vi "Write Pixel Step.vi"(8 "error in (no error)":errorcluster, 10 "Pixel Step":i32, 11 "Listbox Handler in":refnum<class "Listbox Handler.lvclass">) -> (0 "error out":errorcluster, 3 "Listbox Handler out":refnum<class "Listbox Handler.lvclass">)   [LabVIEW 2016, in "Listbox Handler.lvclass"]
uses:
  Listbox Handler.lvclass
  Listbox Handler.lvclass/Listbox Handler.ctl
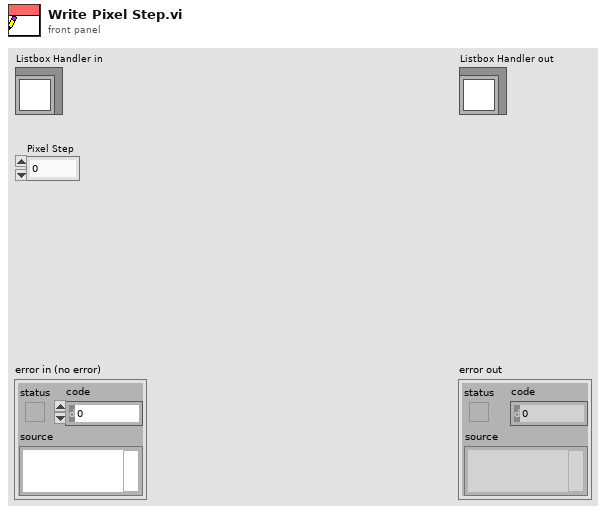
[diagram p1: front panel]
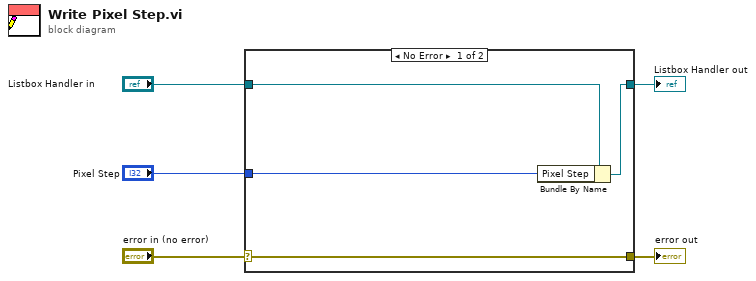
[diagram p0: block diagram]
diagram:
  n1 = case shown="No Error" "error in (no error)" {
    selector: "error in (no error)" -> [w9 w10]
    tunnel: [w9 w10] -> w4
    tunnel: [w7 w11] -> w2
    tunnel: "Listbox Handler in" -> [w8 w11]
    tunnel: "Pixel Step" -> [w6 _]
    frame No Error {
      n2 = Bundle By Name(cluster=w8, "Pixel Step"=w6) -> (w7:refnum<class "Listbox Handler.lvclass">)
    }
    frame Error {
    }
  }
  "error out" <- w4
  "Listbox Handler out" <- w2
